vi "getChannel.vi"(8 "error in (no error)":errorcluster, 10 "index":i32, 11 "ChannelArray.lvclass in":refnum<class "ChannelArray.lvclass">) -> (0 "error out":errorcluster, 2 "Channel":refnum<class "Channel.lvclass">, 3 "ChannelArray.lvclass out":refnum<class "ChannelArray.lvclass">)   [LabVIEW 2011, in "Tools.lvlib" / "DatabaseHelpers.lvlib" / "ChannelArray.lvclass"]
uses:
  ChannelArray.lvclass
  Channel/Channel.lvclass
  ChannelArray.lvclass/ChannelArray.ctl
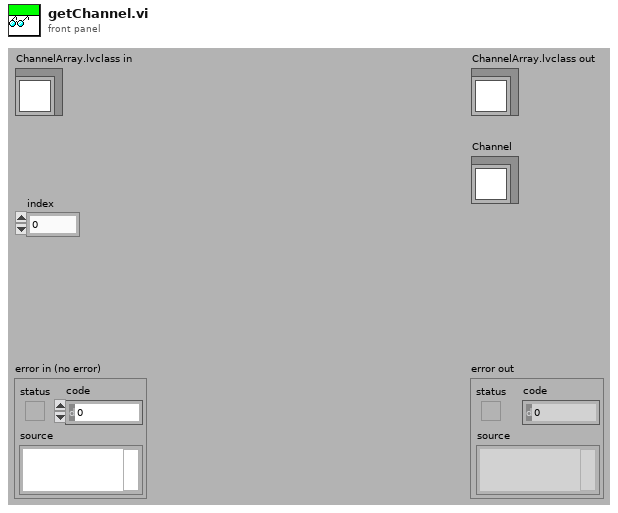
[diagram p1: front panel]
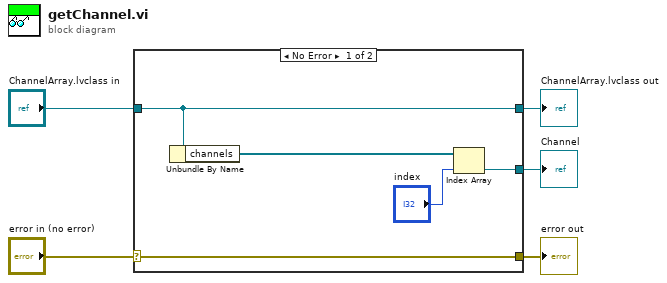
[diagram p0: block diagram]
diagram:
  n1 = case shown="No Error" "error in (no error)" {
    selector: "error in (no error)" -> [w10 w11]
    tunnel: [w10 w11] -> w4
    tunnel: [w9 w12] -> w2
    tunnel: "ChannelArray.lvclass in" -> [w9 w12]
    tunnel: [w6 _] -> w1
    frame No Error {
      n2 = Unbundle By Name(w9) -> ("channels"=w8:refnum<class "Channel.lvclass">[])
      n3 = Index Array(array=w8, index="index") -> (element=w6:refnum<class "Channel.lvclass">)
    }
    frame Error {
    }
  }
  "error out" <- w4
  "ChannelArray.lvclass out" <- w2
  "Channel" <- w1
